vi "Create Mesh.vi"(6 "Draw Mode":T8(ring)=enum."Triangles", 7 "3D Mesh Property":T1={"General Property"={"Plot Name"="", "Coordinate System"=enum."Cartesian", "Opacity"=0.0}, "Projection Property"={"Draw XY"=FALSE, "Draw YZ"=FALSE, "Draw XZ"=FALSE}, "Plot Property"={"Surface Color"=0, "Line Style"=enum."None", "Line Width"=0.0, "Color Ramp Cluster"={"Color Ramp Style"=enum."None", "Color Ramp Array"=[16711934, 393471, 57855, 4390754, 16449346, 16744722, 16711680], "Color Ramp Index"=[45, 91, 133, 175, 219, 255], "Interpolate?"=FALSE, "Logarithm?"=FALSE}, "Antialiasing"=FALSE}, "Mesh Property"={"Mesh Mode"=enum."Lines"}}, 8 "error in (no error)":errorcluster, 9 "Actual Transform In":T7, 10 "Plot Representation In":T4, 11 "Plot Object In":refnum<vi>) -> (0 "error out":errorcluster, 1 "Actual Transform Out":T7, 2 "Plot Representation Out":T4, 3 "Plot Object Out":refnum<vi>, 4 "Mesh Object Out":refnum<vi>)   [LabVIEW 2020, in "3D Mesh.lvclass"]
uses:
  <vilib>/Math Plots/3D Math Plots/3D Mesh/3D Mesh/3D Mesh.lvclass
  <vilib>/Math Plots/3D Math Plots/3D Plot/3D Plot/Typedef/Actual Transform.ctl
  <vilib>/Math Plots/3D Math Plots/3D Plot/3D Plot/Typedef/Range Clusters.ctl
  <vilib>/Math Plots/3D Math Plots/3D Plot/3D Plot/Typedef/Plot Representation.ctl
  <vilib>/Math Plots/3D Math Plots/3D Plot/3D Plot/Typedef/Mesh Data.ctl
  <vilib>/Math Plots/3D Math Plots/3D Mesh/3D Mesh/Typedef/3D Mesh Property.ctl
  <vilib>/Math Plots/3D Math Plots/3D Plot/3D Plot/Typedef/Line Type.ctl
  <vilib>/Math Plots/3D Math Plots/3D Plot/3D Plot/Typedef/Color Ramp Cluster.ctl
  <vilib>/picture/3D Picture Control/NI_3D Picture Control.lvlib
  <vilib>/Math Plots/3D Math Plots/3D Plot/3D Plot/3D Plot.lvclass
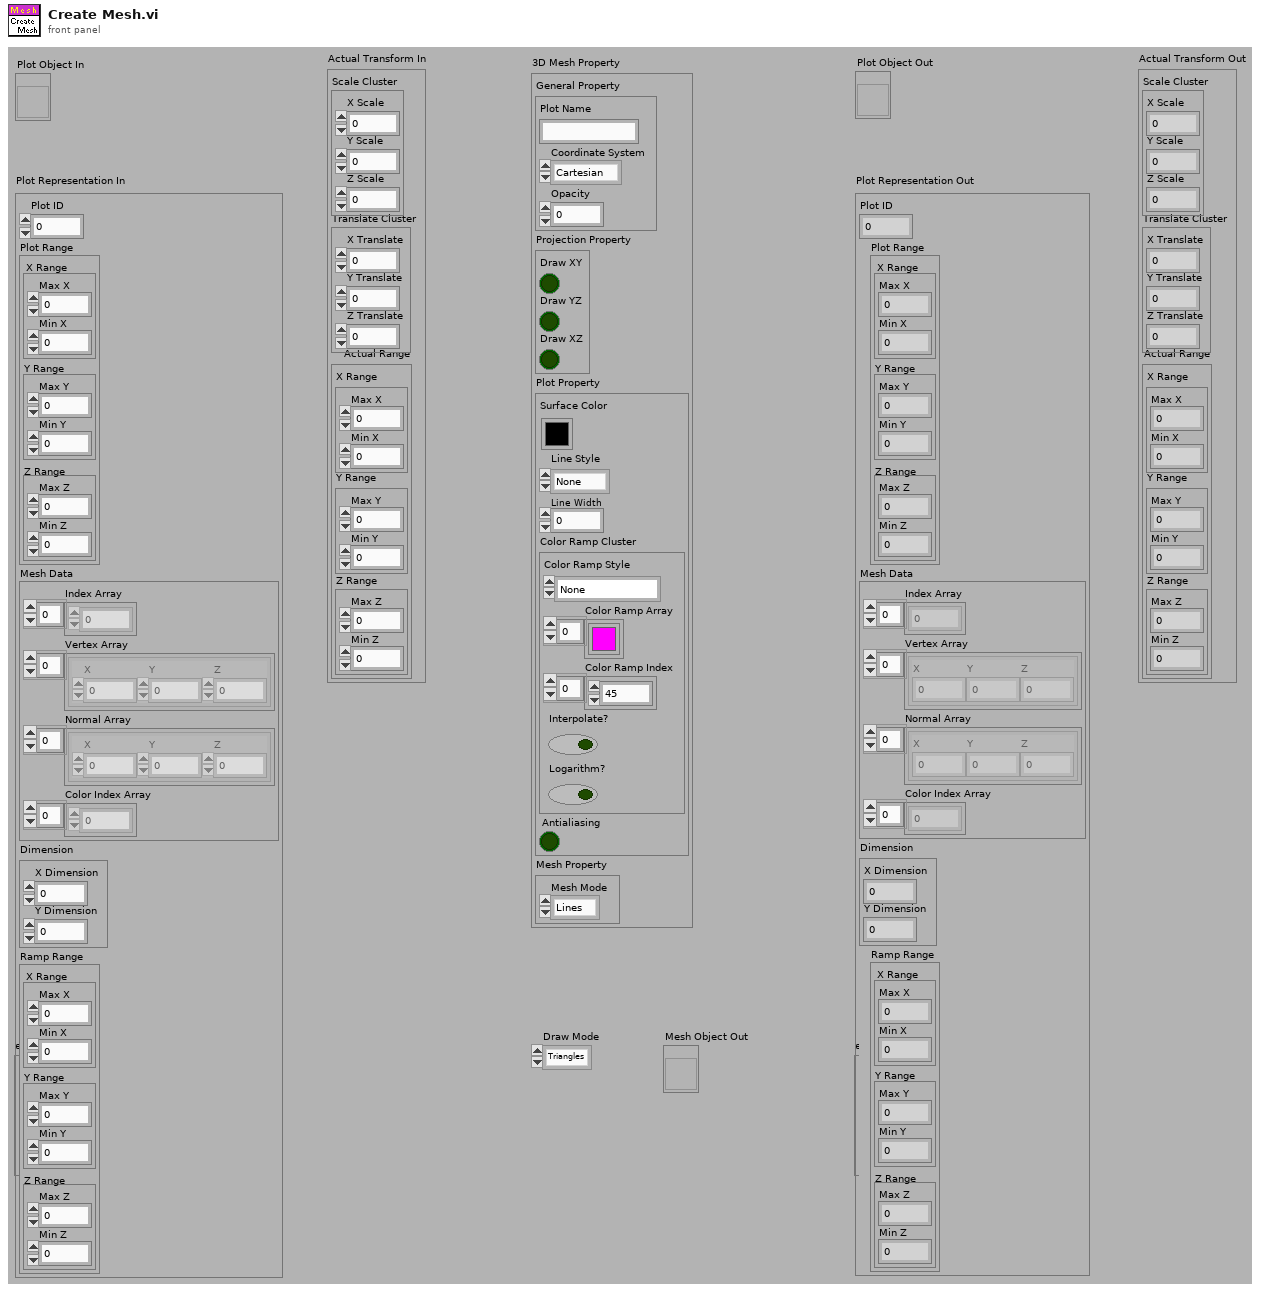
[diagram p1: front panel]
types:
  T1 = typedef "3D Mesh.lvclass/3D Mesh Property.ctl" = cluster{"General Property":cluster{"Plot Name":string, "Coordinate System":enum16{"Cartesian", "Cylindrical", "Spherical"}, "Opacity":sgl}, "Projection Property":cluster{"Draw XY":bool, "Draw YZ":bool, "Draw XZ":bool}, "Plot Property":cluster{"Surface Color":u32, "Line Style":T2, "Line Width":sgl, "Color Ramp Cluster":T3, "Antialiasing":bool}, "Mesh Property":cluster{"Mesh Mode":enum16{"Lines", "Hidden Lines", "With Zero Plane"}}}
  T2 = typedef "3D Plot.lvclass/Line Type.ctl" = enum16{"None", "Solid", "Dash", "Dot", "Dash Dot"}
  T3 = typedef "3D Plot.lvclass/Color Ramp Cluster.ctl" = cluster{"Color Ramp Style":enum16{"None", "Shaded", "Color spectrum", "Grey scale", "Custom"}, "Color Ramp Array":u32[], "Color Ramp Index":i32[], "Interpolate?":bool, "Logarithm?":bool}
  T4 = typedef "3D Plot.lvclass/Plot Representation.ctl" = cluster{"Plot ID":i32, "Plot Range":T5, "Mesh Data":T6, "Dimension":cluster{"X Dimension":i32, "Y Dimension":i32}, "Ramp Range":T5}
  T5 = typedef "3D Plot.lvclass/Range Clusters.ctl" = cluster{"X Range":cluster{"Max X":sgl, "Min X":sgl}, "Y Range":cluster{"Max Y":sgl, "Min Y":sgl}, "Z Range":cluster{"Max Z":sgl, "Min Z":sgl}}
  T6 = typedef "3D Plot.lvclass/Mesh Data.ctl" = cluster{"Index Array":u32[], "Vertex Array":cluster{"X":sgl, "Y":sgl, "Z":sgl}[], "Normal Array":cluster{"X":sgl, "Y":sgl, "Z":sgl}[], "Color Index Array":i32[]}
  T7 = typedef "3D Plot.lvclass/Actual Transform.ctl" = cluster{"Scale Cluster":cluster{"X Scale":sgl, "Y Scale":sgl, "Z Scale":sgl}, "Translate Cluster":cluster{"X Translate":sgl, "Y Translate":sgl, "Z Translate":sgl}, "Actual Range":T5}
  T8 = enum16{"Points", "Lines", "Line Strip", "Line Loop", "Triangles", "Triangle Strip", "Triangle Fan", "Quads", "Quad Strip", "Polygon"}
  T9 = enum16{"Overall", "Per Primitive", "Per Vertex", "Binding Off"}
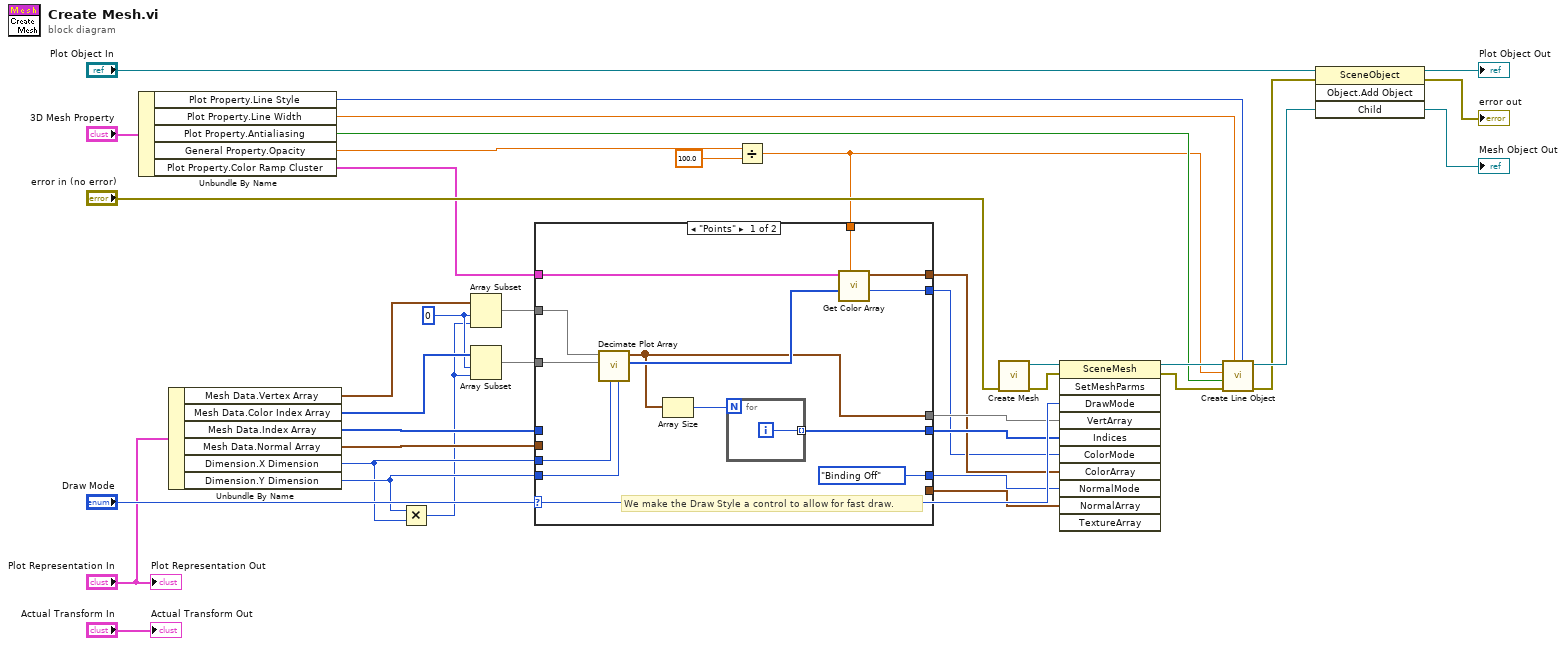
[diagram p0: block diagram]
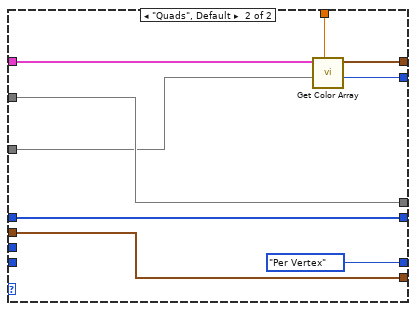
[diagram p2: hidden frame]
diagram:
  w3 = 0 ("length")
  n1 = Unbundle By Name("3D Mesh Property") -> ("Plot Property.Line Style"=w7:T2, "Plot Property.Line Width"=w8:sgl, "Plot Property.Antialiasing"=w5:bool, "General Property.Opacity"=w6:sgl, "Plot Property.Color Ramp Cluster"=w22:T3)
  n2 = Unbundle By Name("Plot Representation In") -> ("Mesh Data.Vertex Array"=w9:cluster{"X":sgl, "Y":sgl, "Z":sgl}[], "Mesh Data.Color Index Array"=w10:i32[], "Mesh Data.Index Array"=w29:u32[], "Mesh Data.Normal Array"=w27:cluster{"X":sgl, "Y":sgl, "Z":sgl}[], "Dimension.X Dimension"=w17:i32, "Dimension.Y Dimension"=w18:i32)
  n3 = Multiply(x=w18, y=w17) -> (x*y=w2:i32)
  n4 = Array Subset(array=w9, index=w3, length=w2) -> (w11:cluster{"X":sgl, "Y":sgl, "Z":sgl}[])
  n5 = Array Subset(array=w10, index=w3, length=w2) -> (w19:i32[])
  n6 = Divide(x=w6, y=sgl 100.0) -> (x/y=w4:sgl)
  n7 = case shown="\"Points\"" "Draw Mode" {
    tunnel: w19 -> [w44 w55]
    tunnel: [w42 w56] -> w24
    tunnel: w29 -> [_ w60]
    tunnel: [w41 w60] -> w28
    tunnel: w27 -> [_ w61]
    tunnel: [_ w61] -> w26
    tunnel: w17 -> [w50 _]
    tunnel: w18 -> [w49 _]
    tunnel: w22 -> [w40 w54]
    tunnel: w4 -> [w46 w57]
    tunnel: [w48 w59] -> w21
    tunnel: [w47 w58] -> w20
    tunnel: w11 -> [w45 w56]
    tunnel: [T9."Binding Off" ("Normal Binding Mode") T9."Per Vertex" ("Normal Binding Mode")] -> w1
    frame "Points" {
      # "We make the Draw Style a control to allow for fast draw."
      n8 = call <vilib>:"Decimate Plot Array.vi"("Y Dimension"=w49, "X Dimension"=w50, "Color Index Array In"=w44, "Vertex Array In"=w45) -> ("Color Index Array Out"=w43:i32[], "Vertex Array Out"=w42:cluster{"X":sgl, "Y":sgl, "Z":sgl}[])  [unwired: 1 in, 5 out]
      n9 = Array Size(array=w42) -> (size(s)=w51:i32)
      n10 = for {
        N: w51 -> [_]
        tunnel: [w52] -> w41 mode=indexing
        i -> [w52]
      }
      n11 = call <vilib>:"Get Color Array.vi"("Alpha"=w46, "Color Index Array"=w43, "Color Ramp Cluster"=w40) -> ("Color Binding Mode"=w47:T9, "Color Array"=w48:cluster{"R":sgl, "G":sgl, "B":sgl, "A":sgl}[])  [unwired: 4 in, 3 out]
    }
    frame "Quads", Default {
      n12 = call <vilib>:"Get Color Array.vi"("Alpha"=w57, "Color Index Array"=w55, "Color Ramp Cluster"=w54) -> ("Color Binding Mode"=w58:T9, "Color Array"=w59:cluster{"R":sgl, "G":sgl, "B":sgl, "A":sgl}[])  [unwired: 4 in, 3 out]
    }
  }
  n13 = call <vilib>:"Create Mesh.vi"("error in (no error)"="error in (no error)") -> ("error out"=w25:errorcluster, "New Mesh Refnum"=w30:refnum<vi>)  [unwired: 9 out]
  n14 = invoke class="SceneMesh" method="SetMeshParms"(reference=w30, error in=w25, "DrawMode"="Draw Mode", "VertArray"=w24, "Indices"=w28, "ColorMode"=w20, "ColorArray"=w21, "NormalMode"=w1, "NormalArray"=w26) -> (reference out=w15:refnum<vi>, error out=w16:errorcluster)  [unwired: 2 in, 9 out]
  n15 = call <vilib>:"Create Line Object.vi"("Line Style"=w7, "Line Width"=w8, "error in (no error)"=w16, "Antialiasing"=w5, "Alpha"=w4, "Mesh Ref In"=w15) -> ("error out"=w12:errorcluster, "Object Ref Out"=w14:refnum<vi>)  [unwired: 4 out]
  n16 = invoke class="SceneObject" method="Object.Add Object"(reference="Plot Object In", error in=w12, "Child"=w14) -> (reference out=→"Plot Object Out":refnum<vi>, error out=→"error out":errorcluster, "Child"=→"Mesh Object Out":refnum<vi>)  [unwired: 1 in, 1 out]
  "Actual Transform Out" <- "Actual Transform In"
  "Plot Representation Out" <- "Plot Representation In"
